vi "findCLFN.vi"(8 "error in (no error)":errorcluster, 10 "vi reference":refnum<vi>, 11 "VI in":refnum<class "VI.lvclass">) -> (0 "error out":errorcluster, 1 "Node Refnum CLFN":refnum<vi>, 2 "found?":bool, 3 "VI out":refnum<class "VI.lvclass">, 4 "Block Diagram":refnum<vi>)   [LabVIEW 2016, in "VI.lvclass"]
uses:
  VI.lvclass
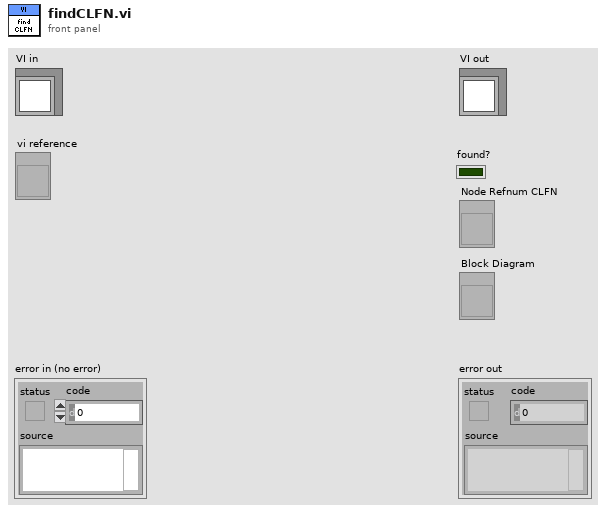
[diagram p1: front panel]
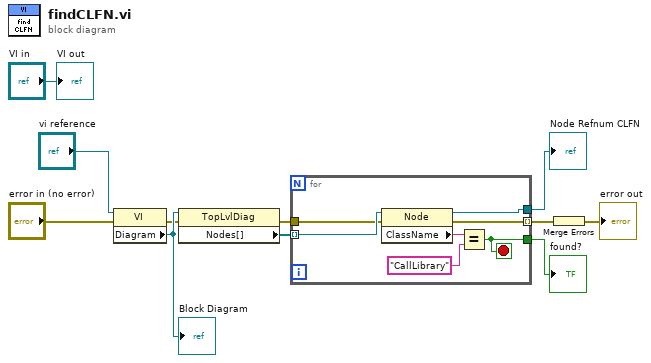
[diagram p0: block diagram]
diagram:
  n1 = property on="Property Node" class="VI"(reference="vi reference", error in="error in (no error)") -> (error out=w6:errorcluster, "Diagram"=w9:refnum<vi>)  [unwired: 1 out]
  "Block Diagram" <- w9
  n2 = property on="Property Node" class="TopLvlDiag"(reference=w9, error in=w6) -> (error out=w5:errorcluster, "Nodes[]"=w10:refnum<vi>[])  [unwired: 1 out]
  n3 = for {
    tunnel: w10 -> [w18] mode=indexing
    tunnel: [w15] -> w1
    tunnel: [w14] -> w8
    tunnel: w5 -> [w13]
    tunnel: [w12] -> w4 mode=indexing
    stop <- w15 stop-if-true
    n4 = property class="Node"(reference=w18, error in=w13) -> (reference out=w14:refnum<vi>, error out=w12:errorcluster, "ClassName"=w17:string)
    n5 = Equal?(x=w17, y="CallLibrary" ("Class Name")) -> (x = y?=w15:bool)
  }
  "Node Refnum CLFN" <- w8
  "found?" <- w1
  n6 = Merge Errors(w4) -> (→"error out":errorcluster)
  "VI out" <- "VI in"
